vi "DO Module to Slot Configuration.vi"(8 "error in":errorcluster, 10 "module in":refnum<class "Module.lvclass">, 11 "slot ref in":T1 format="%.0x") -> (0 "error out":errorcluster, 3 "slot ref out":T1 format="%.0x")   [LabVIEW 2017, in "Scan Engine Scripting.lvlib"]
uses:
  Scan Engine Scripting.lvlib
  <vilib>/NI Veristand/Custom Device API/Custom Device Item Ref.ctl
  Modules/Module/Module.lvclass
  <vilib>/NI Veristand/Custom Device API/Custom Device API.lvlib
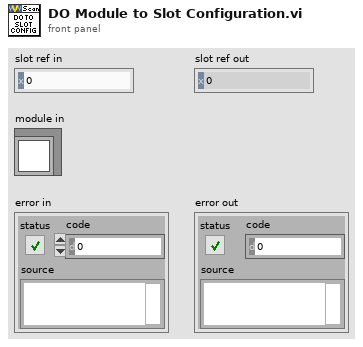
[diagram p1: front panel]
types:
  T1 = typedef "Custom Device API.lvlib/Custom Device Item Ref.ctl" = u64
  T2 = typedef "Scan Engine Scripting.lvlib/digital channel settings.ctl" = cluster{"name":string, "default value":bool}
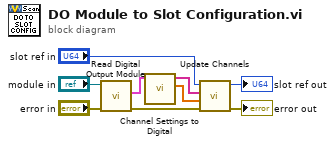
[diagram p0: block diagram]
diagram:
  n1 = call-dynamic "Read Digital Output Module.vi"("error in"="error in", "module in"="module in") -> ("error out"=w4:errorcluster, "channel settings"=w3:T2[])  [unwired: 7 in, 1 out]
  n2 = call "Channel Settings to Digital.vi"("channel settings"=w3) -> ("channel default values"=w9:dbl[], "channel names"=w8:string[])  [unwired: 9 in]
  n3 = call "Update Channels.vi"("error in"=w4, "default values"=w9, "channel names"=w8, "slot ref in"="slot ref in") -> ("error out"=→"error out":errorcluster, "slot ref out"=→"slot ref out":T1)  [unwired: 6 in]
